vi "Calc - TEGTCORR.vi"(7 "PBLimitH":dbl, 9 "PBCOR":dbl, 10 "PBLimitLM":dbl, 11 "TEGT Meas":dbl) -> (2 "TEGTCORRH":dbl, 3 "TEGTCORRLM":dbl)   [LabVIEW 2018, in "Controller (Host).lvlib"]
uses:
  Controller (Host).lvlib
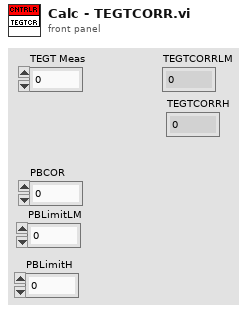
[diagram p1: front panel]
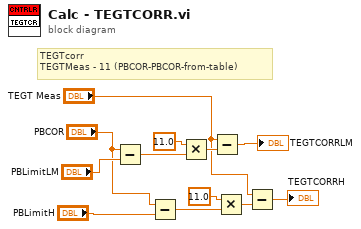
[diagram p0: block diagram]
diagram:
  # "TEGTcorr\nTEGTMeas - 11 (PBCOR-PBCOR-from-table)"
  n1 = Subtract(x="PBCOR", y="PBLimitLM") -> (x-y=w10:dbl)
  n2 = Subtract(x="PBCOR", y="PBLimitH") -> (x-y=w5:dbl)
  n3 = Multiply(x=11.0, y=w10) -> (x*y=w12:dbl)
  n4 = Subtract(x="TEGT Meas", y=w12) -> (x-y=→"TEGTCORRLM":dbl)
  n5 = Multiply(x=11.0, y=w5) -> (x*y=w7:dbl)
  n6 = Subtract(x="TEGT Meas", y=w7) -> (x-y=→"TEGTCORRH":dbl)
